vi "toJSON.vi"(8 "error in (no error)":errorcluster, 11 "tBSONNull in":refnum<class "tBSONNull.lvclass">) -> (0 "error out":errorcluster, 2 "JSON":string, 3 "tBSONNull out":refnum<class "tBSONNull.lvclass">)   [LabVIEW 2013, in "BSON.lvlib" / "tBSONNull.lvclass"]
uses:
  tBSONNull.lvclass
  tBSONElement/tBSONElement.lvclass
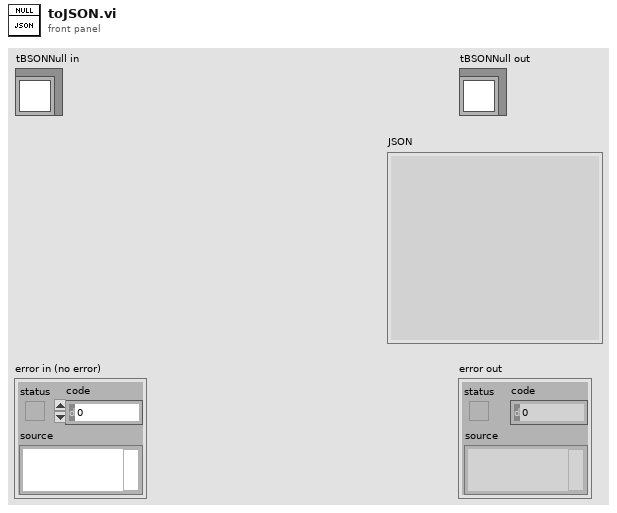
[diagram p1: front panel]
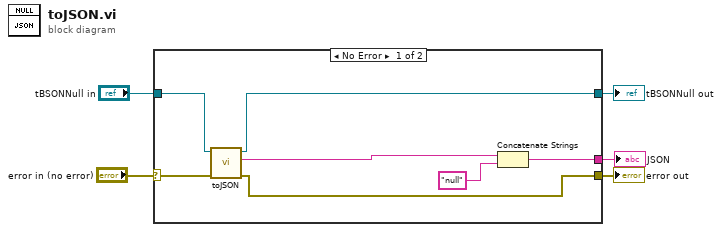
[diagram p0: block diagram]
diagram:
  n1 = case shown="No Error" "error in (no error)" {
    selector: "error in (no error)" -> [w11 w13]
    tunnel: "tBSONNull in" -> [w12 w14]
    tunnel: [w6 w13] -> w2
    tunnel: [w7 w14] -> w4
    tunnel: [w8 _] -> w3
    frame No Error {
      n2 = call-parent "toJSON.vi"("error in (no error)"=w11, "tBSONElement in"=w12) -> ("error out"=w6:errorcluster, "JSON"=w10:string, "tBSONElement out"=w7:refnum<class "tBSONNull.lvclass">)  [unwired: 7 in]
      n3 = Concatenate Strings(w10, "null" ("string")) -> (w8:string)
    }
    frame Error {
    }
  }
  "error out" <- w2
  "tBSONNull out" <- w4
  "JSON" <- w3
